vi "New PropertyContainer.vi"(8 "error in (no error)":errorcluster) -> (0 "error out":errorcluster, 3 "Session Handle out":T1)   [LabVIEW 2020, in "TSS.lvlib" / "VariableContainer.lvclass"]
uses:
  VariableContainer.lvclass
  Typedefs/Session Handle.ctl
  Engine/Engine.lvclass
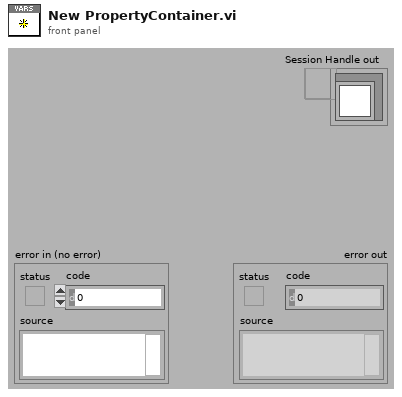
[diagram p1: front panel]
types:
  T1 = typedef "TSS.lvlib/VariableContainer.lvclass/Session Handle.ctl" = refnum<data-value>
  T2 = typedef "TSS.lvlib/Engine.lvclass/Session Handle.ctl" = refnum<data-value>
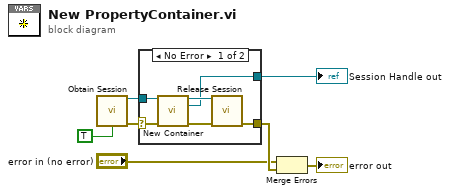
[diagram p0: block diagram]
diagram:
  n1 = call "Obtain Session.vi"("Error to Create? (F)"=TRUE) -> ("Session Handle"=w5:T2, "error out"=w6:errorcluster)  [unwired: 13 in]
  n2 = case shown="No Error" w6 {
    selector: w6 -> [w11 w14]
    tunnel: w5 -> [w12 _]
    tunnel: [w8 _] -> w3
    tunnel: [w13 w14] -> w4
    frame No Error {
      n3 = call "New Container.vi"("Session Handle in"=w12, "error in (no error)"=w11) -> ("Session Handle out"=w9:T2, "New Value Container"=w8:T1, "error out"=w10:errorcluster)  [unwired: 11 in]
      n4 = call "Release Session.vi"("Session Handle"=w9, "error in (no error)"=w10) -> ("error out"=w13:errorcluster)  [unwired: 13 in]
    }
    frame Error {
    }
  }
  "Session Handle out" <- w3
  n5 = Merge Errors("error in (no error)", w4) -> (→"error out":errorcluster)
